vi "Write Supported freq.vi"(10 "Supported freq":cluster{"Minimum":dbl, "Maximum":dbl}, 11 "Vector Network Analyzer in":refnum<class "Vector Network Analyzer.lvclass">) -> (3 "Vector Network Analyzer out":refnum<class "Vector Network Analyzer.lvclass">)   [LabVIEW 2020, in "Vector Network Analyzer.lvclass"]
uses:
  Vector Network Analyzer.lvclass
  Vector Network Analyzer.lvclass/Vector Network Analyzer.ctl
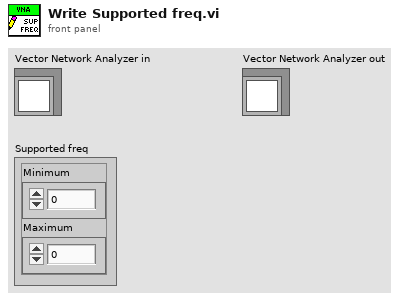
[diagram p1: front panel]
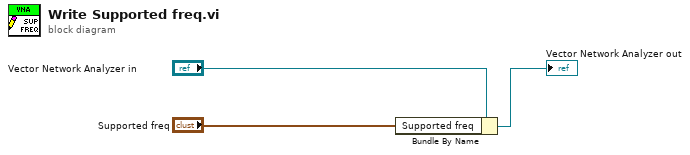
[diagram p0: block diagram]
diagram:
  n1 = Bundle By Name(cluster="Vector Network Analyzer in", "Supported freq"="Supported freq") -> (→"Vector Network Analyzer out":refnum<class "Vector Network Analyzer.lvclass">)
